vi "IHL_Start Collect Helper.vi"(7 "Encoder Cnt":i32, 8 "error in (no error)":errorcluster, 9 "MaxSamples":i32, 10 "PosToEndScan":i32, 11 "EventLog in":refnum<class "EventLog.lvclass">) -> (0 "error out":errorcluster, 1 "Success":bool, 2 "data value reference":refnum<data-value>, 3 "Block Cnt notifier out":refnum<notifier>)   [LabVIEW 2015, in "Tool Module.lvlib"]
uses:
  Tool Module.lvlib
  Event Logger Library/Event Log/EventLog.lvclass
  Collect Data Mgr/Data Collect Parameters typedef--cluster.ctl
  Tool Interface/_HS Data Stream Params Cluster--typedef.ctl
  Collect Data Mgr/Start Collect (Reply Payload)--cluster.ctl
  ToolModGLOB.vi
  Tool Config/Tool Cfg.lvlib
  Collect Data Mgr/Collect Data Mgr.lvlib
  Tool Interface/Tool Interface.lvlib
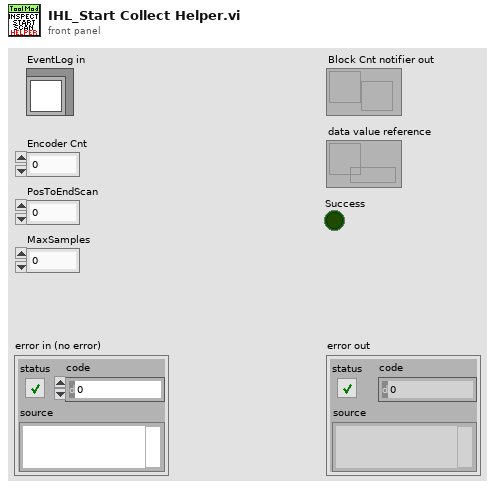
[diagram p1: front panel]
types:
  T1 = typedef "Collect Data Mgr.lvlib/Start Collect (Reply Payload)--cluster.ctl" = cluster{"Success":bool, "CD_Status":u8}
  T2 = enum16{"Idle", "Receive HS Data", "Close Connection"}
  T3 = typedef "Tool Interface.lvlib/_HS Data Stream Params Cluster--typedef.ctl" = cluster{"Raw Data Stream Loop cmd":enum16{"Idle", "Receive HS Data", "Close Connection"}, "Data Array DVR ref":refnum<data-value>, "Sample Data notifier":refnum<notifier>, "Block Count Notifier":refnum<notifier>}
  T4 = typedef "Collect Data Mgr.lvlib/Data Collect Parameters typedef--cluster.ctl" = cluster{"Mode":i8, "Move Length":i32, "Array Length":i32, "Max Samples":i32}
  T5 = typedef "Tool Cfg.lvlib/_Tool Operation Config Cluster--typedef.ctl" = cluster{"Use Tool Cfg":bool, "Use Tool Cal":bool, "Fake Data?":bool, "Mode":i16, "Array Subset Length":i16, "nArrays to Read":i16, "Full Array Read Length":i16, "nSubarrays/Sensor":i16}
  T6 = typedef "_Data Stream Fmt Params Cluster--typedef.ctl" = cluster{"Samples per Block":i32, "Raw Data Status Len":i32, "Fltr Data Status Len":i32}
  T7 = typedef "Tool Interface.lvlib/_Loop Ctrl Notifiers Cluster--typedef.ctl" = cluster{"Raw Stream Ctrl":refnum<notifier>}
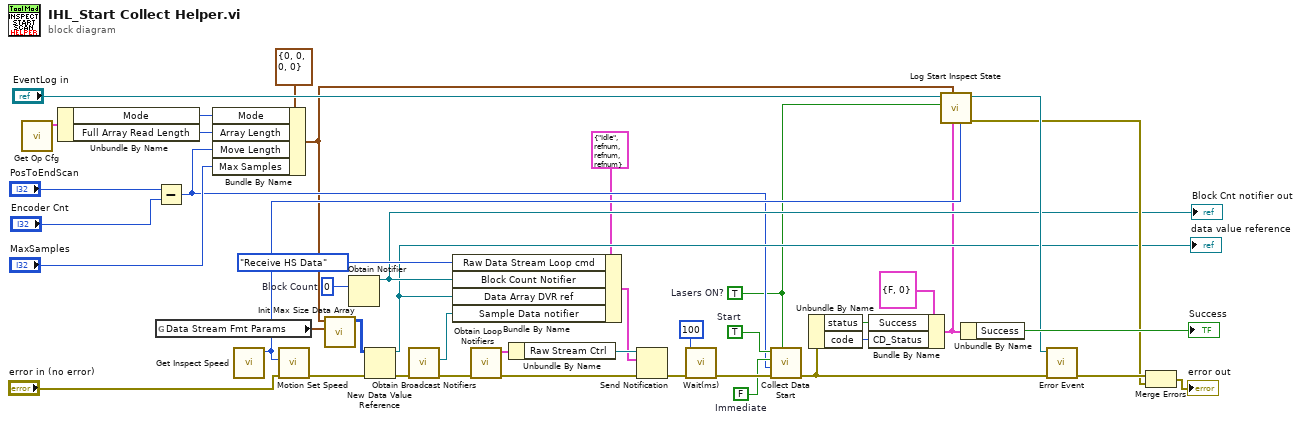
[diagram p0: block diagram]
diagram:
  w12 = FALSE  # Immediate
  w11 = TRUE  # Start
  w21 = u32 0  # Block Count
  w4 = TRUE  # Lasers ON?
  n1 = call "Get Op Cfg.vi"() -> ("Tool Operation Config"=w39:T5)  [unwired: 11 in]
  n2 = Unbundle By Name(w39) -> ("Mode"=w38:i16, "Full Array Read Length"=w37:i16)
  n3 = Subtract(x="PosToEndScan", y="Encoder Cnt") -> (x-y=w10:i32)
  n4 = global read "ToolModGLOB.vi" "Data Stream Fmt Params"() -> (w33:T6)
  n5 = Bundle By Name(cluster=T4 {"Mode"=0, "Move Length"=0, "Array Length"=0, "Max Samples"=0} ("_Data Collect Params typedef--cluster"), "Mode"=w38, "Array Length"=w37, "Move Length"=w10, "Max Samples"="MaxSamples") -> (w3:T4)
  n6 = call "Get Inspect Speed.vi"() -> ("Inspect Speed"=w40:u16)  [unwired: 11 in]
  n7 = call "Motion Set Speed.vi"("error in (no error)"="error in (no error)", "Speed"=w40) -> ("error out"=w31:errorcluster)  [unwired: 9 in]
  n8 = call "Init Max Size Data Array.vi"("Data Stream Fmt Params"=w33, "Data Collect Params"=w3) -> ("initialized array"=w32:u32[][])  [unwired: 9 in]
  n9 = Obtain Notifier(notification data type=w21) -> (notifier out=w20:refnum<notifier>)  [unwired: 3 in, 2 out]
  "Block Cnt notifier out" <- w20
  n10 = New Data Value Reference(data value=w32, error in=w31) -> (data value reference=w16:refnum<data-value>, error out=w19:errorcluster)
  "data value reference" <- w16
  n11 = call "Obtain Broadcast Notifiers.vi"("error in (no error)"=w19) -> ("error out"=w1:errorcluster, "Sample Data notifier out"=w15:refnum<notifier>)  [unwired: 9 in]
  n12 = Bundle By Name(cluster=T3 {"Raw Data Stream Loop cmd"=enum."Idle", "Data Array DVR ref"=refnum, "Sample Data notifier"=refnum, "Block Count Notifier"=refnum} ("Cluster"), "Raw Data Stream Loop cmd"=T2."Receive HS Data" ("HS Data Stream SM enum"), "Block Count Notifier"=w20, "Data Array DVR ref"=w16, "Sample Data notifier"=w15) -> (w17:T3)
  n13 = call "Obtain Loop Notifiers.vi"("error in (no error)"=w1) -> ("error out"=w18:errorcluster, "Loop Ctrl Notifiers Cluster"=w23:T7)  [unwired: 9 in]
  n14 = Unbundle By Name(w23) -> ("Raw Stream Ctrl"=w22:refnum<notifier>)
  n15 = Send Notification(notification=w17, notifier=w22, error in (no error)=w18) -> (error out=w13:errorcluster)  [unwired: 1 out]
  n16 = call "Wait(ms).vi"("error in (no error)"=w13, "milliseconds"=u32 100) -> ("error out"=w42:errorcluster)  [unwired: 9 in]
  n17 = call "Collect Data Start.vi"("Lasers ON?"=w4, "error in (no error)"=w42, "Length"=w10, "Immediate"=w12, "Start"=w11) -> ("error out"=w5:errorcluster)  [unwired: 6 in]
  n18 = Unbundle By Name(w5) -> ("status"=w9:bool, "code"=w7:i32)
  n19 = Bundle By Name(cluster=T1 {"Success"=FALSE, "CD_Status"=0} ("Start Collect (Reply Payload)"), "Success"=w9, "CD_Status"=w7) -> (w6:T1)
  n20 = call "Log Start Inspect State.vi"("Speed"=w40, "Start Collect (Reply Payload)"=w6, "Data Collect Params"=w3, "Laser On"=w4, "EventLog in"="EventLog in") -> ("error out"=w25:errorcluster, "EventLog out"=w29:refnum<class "EventLog.lvclass">)  [unwired: 5 in]
  n21 = Unbundle By Name(w6) -> ("Success"=→"Success":bool)
  n22 = call "Error Event.vi"("error in (no error)"=w5, "EventLog ref"=w29) -> ("error out"=w26:errorcluster)  [unwired: 8 in, 1 out]
  n23 = Merge Errors(w26, w25) -> (→"error out":errorcluster)
